vi "Comm Connect.vi"(8 "error in (no error)":errorcluster, 11 "niDTS Comm Serial in":refnum<class "niDTS Comm Serial.lvclass">) -> (0 "error out":errorcluster, 3 "niDTS Comm Serial out":refnum<class "niDTS Comm Serial.lvclass">)   [LabVIEW 2015, in "niDTS CommLib.lvlib" / "niDTS Comm Serial.lvclass"]
uses:
  niDTS Comm Serial.lvclass
  Framework/Logger/Includes/niDTS Logger INC Log Element Type.ctl
  Dependencies/__VISA Configure Serial Port (Instr).vi
  Framework/Logger/Objects/BASE_class/niDTS Logger.lvclass
  Framework/niDTS Framework.lvlib
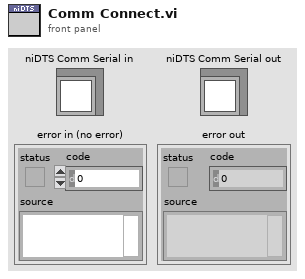
[diagram p1: front panel]
types:
  T1 = typedef "niDTS Framework.lvlib/niDTS Logger INC Log Element Type.ctl" = enum16{"Error", "Warning", "Information", "Debugging"}
  T2 = cluster{"baud rate ":u32, "data bits":u16, "Enable Termination Char":bool, "flow control":u16, "parity":enum16{"None", "Odd", "Even", "Mark", "Space"}, "timeout (ms) ":u32, "stop bits":u16, "termination char":u8}
  T3 = typedef "niDTS Framework.lvlib/niDTS Logger INC Handle.ctl" = refnum<data-value>
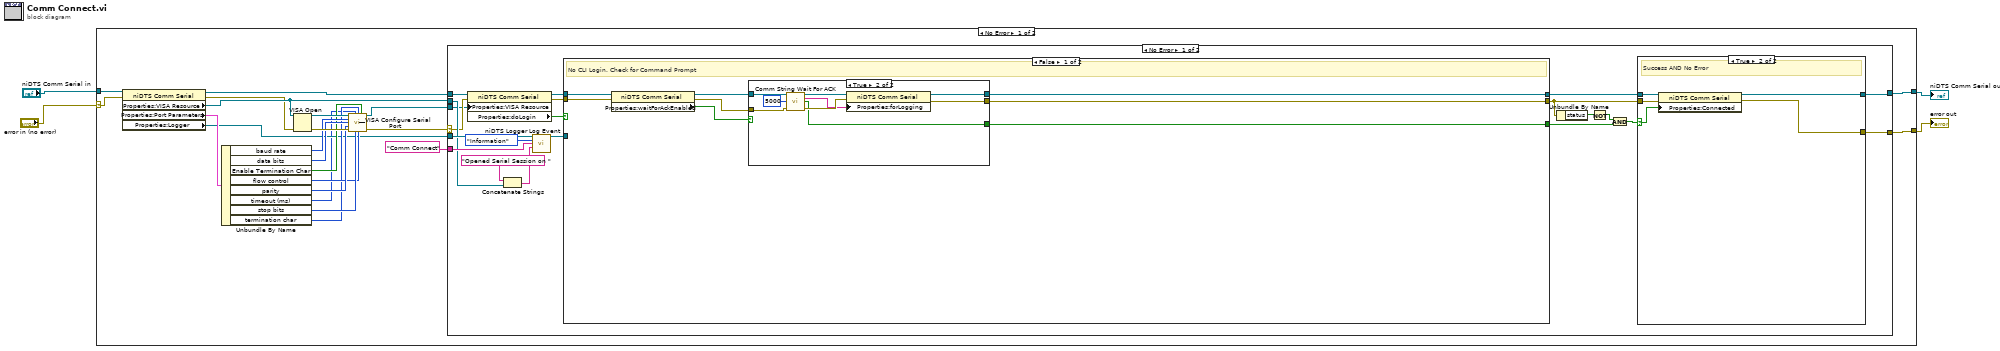
[diagram p0: block diagram]
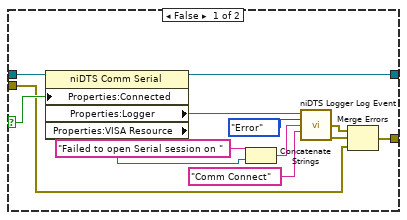
[diagram p2: hidden frame]
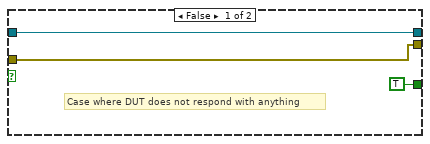
[diagram p3: hidden frame]
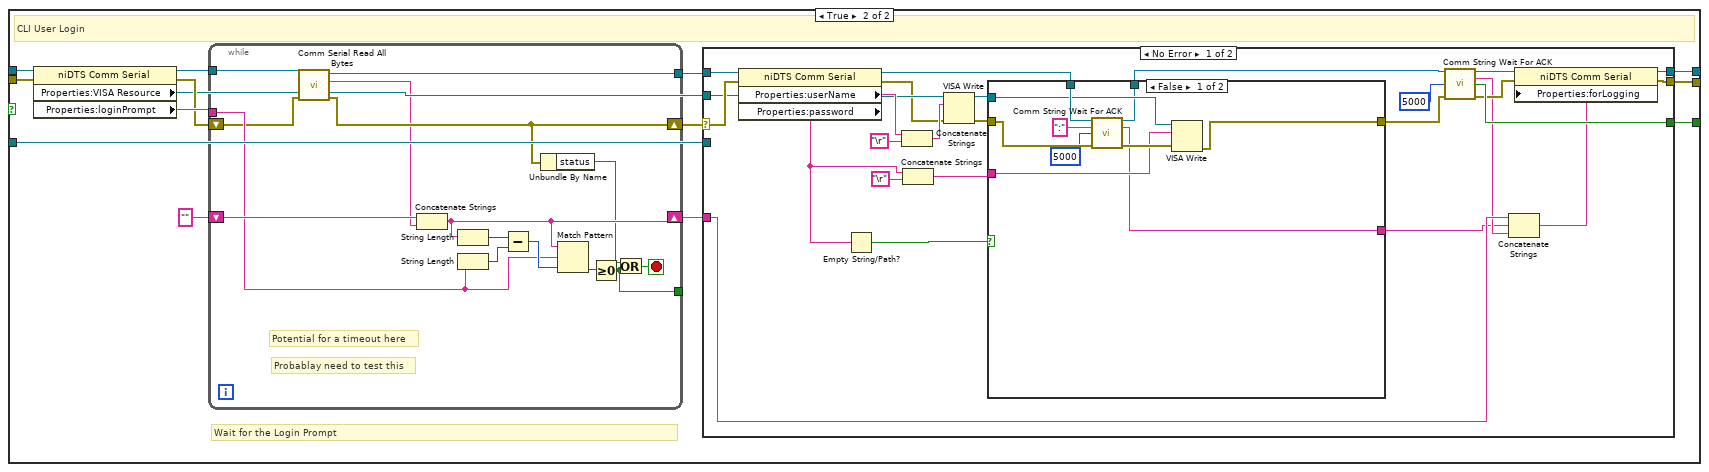
[diagram p4: hidden frame]
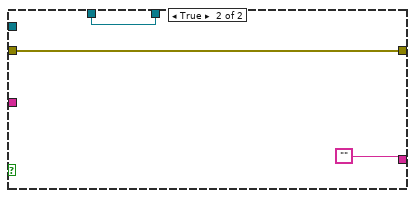
[diagram p5: hidden frame]
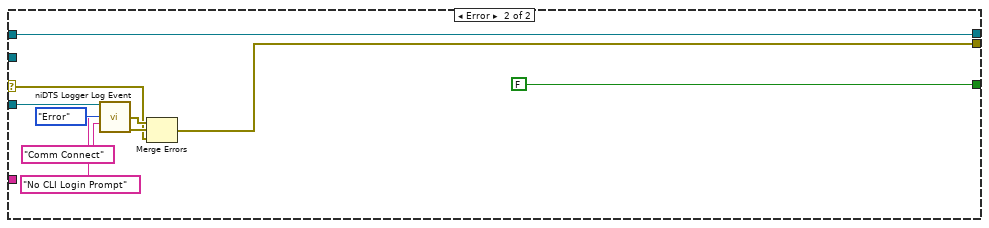
[diagram p6: hidden frame]
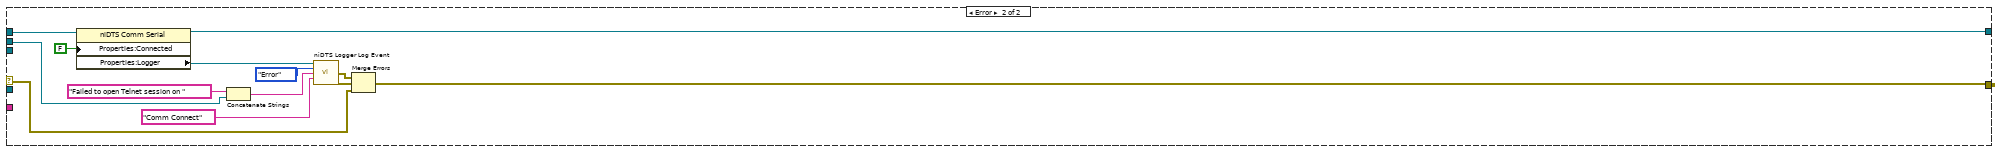
[diagram p7: hidden frame]
diagram:
  n1 = case shown="No Error" "error in (no error)" {
    selector: "error in (no error)" -> [w24 w177]
    tunnel: "niDTS Comm Serial in" -> [w26 w178]
    tunnel: [w22 w178] -> w2
    tunnel: [w20 w177] -> w1
    frame No Error {
      n2 = property class="niDTS Comm Serial"(reference=w26, error in=w24) -> (reference out=w23:refnum<class "niDTS Comm Serial.lvclass">, error out=w18:errorcluster, "Properties:VISA Resource"=w19:refnum<visa-resource-name>, "Properties:Port Parameters"=w25:T2, "Properties:Logger"=w7:T3)
      n3 = Unbundle By Name(w25) -> ("baud rate"=w14:u32, "data bits"=w13:u16, "Enable Termination Char"=w8:bool, "flow control"=w10:u16, "parity"=w12:enum16{"None", "Odd", "Even", "Mark", "Space"}, "timeout (ms)"=w6:u32, "stop bits"=w11:u16, "termination char"=w9:u8)
      n4 = VISA Open(error in (no error)=w18, VISA resource name=w19) -> (VISA resource name=w17:refnum<visa-resource-name>, error out=w16:errorcluster)  [unwired: 3 in]
      n5 = call-poly "__VISA Configure Serial Port"("VISA resource name"=w17, "timeout (10sec)"=w6, "termination char\n(0xA = '\\n' = LF)"=w9, "Enable Termination\nChar (T)"=w8, "baud rate (9600)"=w14, "data bits (8)"=w13, "parity (0:none)"=w12, "error in (no error)"=w16, "stop bits (10: 1 bit)"=w11, "flow control (0:none)"=w10) -> ("VISA resource name out"=w5:refnum<visa-resource-name>, "error out"=w15:errorcluster)  [unwired: 4 in]
      n6 = case shown="No Error" w15 {
        selector: w15 -> [w40 w166]
        tunnel: w5 -> [w39 _]
        tunnel: w23 -> [w41 w176]
        tunnel: w19 -> [w43 w169]
        tunnel: [w27 w165] -> w20
        tunnel: [w28 w164] -> w22
        tunnel: w7 -> [w47 _]
        tunnel: "Comm Connect" ("Description/Data") -> [w45 _]
        frame No Error {
          n7 = property class="niDTS Comm Serial"(reference=w41, error in=w40, "Properties:VISA Resource"=w39) -> (reference out=w37:refnum<class "niDTS Comm Serial.lvclass">, error out=w36:errorcluster, "Properties:doLogin"=w38:bool)
          n8 = Concatenate Strings("Opened Serial Session on ", w43) -> (w42:string)
          n9 = call "niDTS Logger Log Event.vi"("Logger Handle"=w47, "Type"=niDTS_Logger_INC_Log_Element_Type."Information", "Description/Data"=w45, "Source/Location"=w42) -> ("Logger Handle out"=w35:T3)  [unwired: 9 in, 2 out]
          n10 = case shown="False" w38 {
            tunnel: w37 -> [w68 w99]
            tunnel: w36 -> [w73 w98]
            tunnel: w35 -> [_ w93]
            tunnel: [w72 w91] -> w34
            tunnel: [w71 w90] -> w30
            tunnel: [w70 w89] -> w29
            frame False {
              # "No CLI Login. Check for Command Prompt"
              n11 = property class="niDTS Comm Serial"(reference=w68, error in=w73) -> (reference out=w67:refnum<class "niDTS Comm Serial.lvclass">, error out=w69:errorcluster, "Properties:waitForAckEnabled"=w66:bool)
              n12 = case shown="True" w66 {
                tunnel: w67 -> [w76 w84]
                tunnel: w69 -> [w75 w82]
                tunnel: [TRUE ("Sucess") w79] -> w72
                tunnel: [w76 w78] -> w71
                tunnel: [w75 w77] -> w70
                frame False {
                  # "Case where DUT does not respond with anything"
                }
                frame True {
                  n13 = call-dynamic "Comm String Wait For ACK.vi"("niDTS Comm Serial in"=w84, "Timeout (ms)"=5000, "error in (no error)"=w82) -> ("niDTS Comm Serial out"=w83:refnum<class "niDTS Comm Serial.lvclass">, "Response"=w80:string, "Sucess"=w79:bool, "error out"=w81:errorcluster)  [unwired: 9 in]
                  n14 = property class="niDTS Comm Serial"(reference=w83, error in=w81, "Properties:forLogging"=w80) -> (reference out=w78:refnum<class "niDTS Comm Serial.lvclass">, error out=w77:errorcluster)
                }
              }
            }
            frame True {
              # "Wait for the Login Prompt"
              # "CLI User Login"
              n15 = property class="niDTS Comm Serial"(reference=w99, error in=w98) -> (reference out=w88:refnum<class "niDTS Comm Serial.lvclass">, error out=w95:errorcluster, "Properties:VISA Resource"=w86:refnum<visa-resource-name>, "Properties:loginPrompt"=w96:string)
              n16 = while "Wait for the login prompt" {
                shift-right: [w158] -> w92
                shift-left: "" -> [w163]
                shift-right: [w150] -> w94
                shift-left: w95 -> [w151]
                tunnel: w96 -> [w157]
                tunnel: [w154] -> _
                tunnel: w88 -> [w153]
                tunnel: [w152] -> w87
                stop <- w155 stop-if-true
                # "Probablay need to test this"
                # "Potential for a timeout here"
                n17 = call-dynamic "Comm Serial Read All Bytes.vi"("error in (no error)"=w151, "niDTS Comm Serial in"=w153) -> ("error out"=w150:errorcluster, "Read"=w149:string, "niDTS Comm Serial out"=w152:refnum<class "niDTS Comm Serial.lvclass">)  [unwired: 7 in]
                n18 = Concatenate Strings(w163, w149) -> (w158:string)
                n19 = String Length(string=w158) -> (length=w161:i32)
                n20 = String Length(string=w157) -> (length=w160:i32)
                n21 = Subtract(x=w161, y=w160) -> (x-y=w159:i32)
                n22 = Unbundle By Name(w150) -> ("status"=w156:bool)
                n23 = Match Pattern(string=w158, regular expression=w157, offset (0)=w159) -> (offset past match=w162:i32)  [unwired: 3 out]
                n24 = Greater Or Equal To 0?(x=w162) -> (x >= 0?=w154:bool)
                n25 = Or(x=w156, y=w154) -> (x .or. y?=w155:bool)
              }
              n26 = case shown="No Error" w94 {
                selector: w94 -> [w124 w140]
                tunnel: w86 -> [w103 _]
                tunnel: w87 -> [w125 w141]
                tunnel: w93 -> [_ w143]
                tunnel: [w122 FALSE ("Sucess")] -> w91
                tunnel: w92 -> [w116 _]
                tunnel: [w118 w141] -> w90
                tunnel: [w117 w139] -> w89
                frame No Error {
                  n27 = property class="niDTS Comm Serial"(reference=w125, error in=w124) -> (reference out=w113:refnum<class "niDTS Comm Serial.lvclass">, error out=w102:errorcluster, "Properties:userName"=w109:string, "Properties:password"=w106:string)
                  n28 = Empty String/Path?(string/path=w106) -> (empty?=w115:bool)
                  n29 = Concatenate Strings(w109, "\r") -> (w104:string)
                  n30 = Concatenate Strings(w106, "\r") -> (w105:string)
                  n31 = VISA Write(VISA resource name=w103, write buffer=w104, error in (no error)=w102) -> (VISA resource name out=w101:refnum<visa-resource-name>, error out=w100:errorcluster)  [unwired: 1 out]
                  n32 = case shown="False" w115 {
                    tunnel: w100 -> [w133 w138]
                    tunnel: [w128 w138] -> w114
                    tunnel: w113 -> [w135 w137]
                    tunnel: w101 -> [w132 _]
                    tunnel: w105 -> [w130 _]
                    tunnel: [w129 w137] -> w112
                    tunnel: [w127 ""] -> w110
                    frame False {
                      n33 = call-dynamic "Comm String Wait For ACK.vi"("niDTS Comm Serial in"=w135, "ACK"=":", "Timeout (ms)"=5000, "error in (no error)"=w133) -> ("niDTS Comm Serial out"=w129:refnum<class "niDTS Comm Serial.lvclass">, "Response"=w127:string, "error out"=w131:errorcluster)  [unwired: 8 in, 1 out]
                      n34 = VISA Write(VISA resource name=w132, write buffer=w130, error in (no error)=w131) -> (error out=w128:errorcluster)  [unwired: 2 out]
                    }
                    frame True {
                    }
                  }
                  n35 = call-dynamic "Comm String Wait For ACK.vi"("niDTS Comm Serial in"=w112, "Timeout (ms)"=5000, "error in (no error)"=w114) -> ("niDTS Comm Serial out"=w121:refnum<class "niDTS Comm Serial.lvclass">, "Response"=w111:string, "Sucess"=w122:bool, "error out"=w120:errorcluster)  [unwired: 9 in]
                  n36 = Concatenate Strings(w116, w110, w111) -> (w119:string)
                  n37 = property class="niDTS Comm Serial"(reference=w121, error in=w120, "Properties:forLogging"=w119) -> (reference out=w118:refnum<class "niDTS Comm Serial.lvclass">, error out=w117:errorcluster)
                }
                frame Error {
                  n38 = call "niDTS Logger Log Event.vi"("Logger Handle"=w143, "Type"=niDTS_Logger_INC_Log_Element_Type."Error", "Description/Data"="No CLI Login Prompt", "Source/Location"="Comm Connect" ("Description/Data")) -> ("Source Data Error"=w146:errorcluster, "error out"=w147:errorcluster)  [unwired: 9 in, 1 out]
                  n39 = Merge Errors(w146, w147, w140) -> (w139:errorcluster)
                }
              }
            }
          }
          n40 = Unbundle By Name(w29) -> ("status"=w32:bool)
          n41 = Not(x=w32) -> (.not. x?=w33:bool)
          n42 = And(x=w33, y=w34) -> (x .and. y?=w31:bool)
          n43 = case shown="True" w31 {
            selector: w31 -> [w59 w63]
            tunnel: w30 -> [w60 w65]
            tunnel: w29 -> [w51 w64]
            tunnel: [w50 w62] -> w28
            tunnel: [w49 w61] -> w27
            frame False {
              n44 = property class="niDTS Comm Serial"(reference=w60, "Properties:Connected"=w59) -> (reference out=w50:refnum<class "niDTS Comm Serial.lvclass">, "Properties:Logger"=w52:T3, "Properties:VISA Resource"=w48:refnum<visa-resource-name>)  [unwired: 1 in, 1 out]
              n45 = Concatenate Strings("Failed to open Serial session on " ("string"), w48) -> (w56:string)
              n46 = call "niDTS Logger Log Event.vi"("Logger Handle"=w52, "Type"=niDTS_Logger_INC_Log_Element_Type."Error", "Description/Data"=w56, "Source/Location"="Comm Connect") -> ("Source Data Error"=w55:errorcluster, "error out"=w54:errorcluster)  [unwired: 9 in, 1 out]
              n47 = Merge Errors(w55, w54, w51) -> (w49:errorcluster)
            }
            frame True {
              # "Success AND No Error"
              n48 = property class="niDTS Comm Serial"(reference=w65, error in=w64, "Properties:Connected"=w63) -> (reference out=w62:refnum<class "niDTS Comm Serial.lvclass">, error out=w61:errorcluster)
            }
          }
        }
        frame Error {
          n49 = property class="niDTS Comm Serial"(reference=w176, "Properties:Connected"=FALSE ("Connected")) -> (reference out=w164:refnum<class "niDTS Comm Serial.lvclass">, "Properties:Logger"=w171:T3)  [unwired: 1 in, 1 out]
          n50 = Concatenate Strings("Failed to open Telnet session on " ("string"), w169) -> (w168:string)
          n51 = call "niDTS Logger Log Event.vi"("Logger Handle"=w171, "Type"=niDTS_Logger_INC_Log_Element_Type."Error", "Description/Data"=w168, "Source/Location"="Comm Connect") -> ("Source Data Error"=w172:errorcluster, "error out"=w173:errorcluster)  [unwired: 9 in, 1 out]
          n52 = Merge Errors(w172, w173, w166) -> (w165:errorcluster)
        }
      }
    }
    frame Error {
    }
  }
  "error out" <- w1
  "niDTS Comm Serial out" <- w2
